vi "get iGPS result.vi"(8 "error in":errorcluster, 10 "serial number":string, 11 "PLC Comms":T3={"PLC boolean read Tags"={"AT glass position"={"Tag Name"="S060.PXI.Signals.PlltData.SN", "Network Path"="172.15.51.1,1,0", "use opc"=FALSE, "DataSocket Reference"={"CWDSLib._DCWDataSocket"=refnum, "CWDSLib._DCWData"=refnum, "OnDataUpdated"=0, "OnStatusUpdated"=0}}, "AT shade position"={"Tag Name"="S060.PXI.Signals.PlltData.SN", "Network Path"="172.15.51.1,1,0", "use opc"=FALSE, "DataSocket Reference"={"CWDSLib._DCWDataSocket"=refnum, "CWDSLib._DCWData"=refnum, "OnDataUpdated"=0, "OnStatusUpdated"=0}}, "AT in glass wand lower pos"={"Tag Name"="S060.PXI.Signals.PlltData.SN", "Network Path"="172.15.51.1,1,0", "use opc"=FALSE, "DataSocket Reference"={"CWDSLib._DCWDataSocket"=refnum, "CWDSLib._DCWData"=refnum, "OnDataUpdated"=0, "OnStatusUpdated"=0}}, "AT in sunshad wand lower pos"={"Tag Name"="S060.PXI.Signals.PlltData.SN", "Network Path"="172.15.51.1,1,0", "use opc"=FALSE, "DataSocket Reference"={"CWDSLib._DCWDataSocket"=refnum, "CWDSLib._DCWData"=refnum, "OnDataUpdated"=0, "OnStatusUpdated"=0}}, "AT in wand home pos"={"Tag Name"="S060.PXI.Signals.PlltData.SN", "Network Path"="172.15.51.1,1,0", "use opc"=FALSE, "DataSocket Reference"={"CWDSLib._DCWDataSocket"=refnum, "CWDSLib._DCWData"=refnum, "OnDataUpdated"=0, "OnStatusUpdated"=0}}, "LVDT's Extended"={"Tag Name"="S060.PXI.Signals.PlltData.SN", "Network Path"="172.15.51.1,1,0", "use opc"=FALSE, "DataSocket Reference"={"CWDSLib._DCWDataSocket"=refnum, "CWDSLib._DCWData"=refnum, "OnDataUpdated"=0, "OnStatusUpdated"=0}}, "bolt check 1"={"Tag Name"="S060.PXI.Signals.PlltData.SN", "Network Path"="172.15.51.1,1,0", "use opc"=FALSE, "DataSocket Reference"={"CWDSLib._DCWDataSocket"=refnum, "CWDSLib._DCWData"=refnum, "OnDataUpdated"=0, "OnStatusUpdated"=0}}, "bolt check 2"={"Tag Name"="S060.PXI.Signals.PlltData.SN", "Network Path"="172.15.51.1,1,0", "use opc"=FALSE, "DataSocket Reference"={"CWDSLib._DCWDataSocket"=refnum, "CWDSLib._DCWData"=refnum, "OnDataUpdated"=0, "OnStatusUpdated"=0}}, "bolt check 3"={"Tag Name"="S060.PXI.Signals.PlltData.SN", "Network Path"="172.15.51.1,1,0", "use opc"=FALSE, "DataSocket Reference"={"CWDSLib._DCWDataSocket"=refnum, "CWDSLib._DCWData"=refnum, "OnDataUpdated"=0, "OnStatusUpdated"=0}}, "bolt check 4"={"Tag Name"="S060.PXI.Signals.PlltData.SN", "Network Path"="172.15.51.1,1,0", "use opc"=FALSE, "DataSocket Reference"={"CWDSLib._DCWDataSocket"=refnum, "CWDSLib._DCWData"=refnum, "OnDataUpdated"=0, "OnStatusUpdated"=0}}, "bolt check 5"={"Tag Name"="S060.PXI.Signals.PlltData.SN", "Network Path"="172.15.51.1,1,0", "use opc"=FALSE, "DataSocket Reference"={"CWDSLib._DCWDataSocket"=refnum, "CWDSLib._DCWData"=refnum, "OnDataUpdated"=0, "OnStatusUpdated"=0}}, "bolt check 6"={"Tag Name"="S060.PXI.Signals.PlltData.SN", "Network Path"="172.15.51.1,1,0", "use opc"=FALSE, "DataSocket Reference"={"CWDSLib._DCWDataSocket"=refnum, "CWDSLib._DCWData"=refnum, "OnDataUpdated"=0, "OnStatusUpdated"=0}}, "bolt check 7"={"Tag Name"="S060.PXI.Signals.PlltData.SN", "Network Path"="172.15.51.1,1,0", "use opc"=FALSE, "DataSocket Reference"={"CWDSLib._DCWDataSocket"=refnum, "CWDSLib._DCWData"=refnum, "OnDataUpdated"=0, "OnStatusUpdated"=0}}, "bolt check 8"={"Tag Name"="S060.PXI.Signals.PlltData.SN", "Network Path"="172.15.51.1,1,0", "use opc"=FALSE, "DataSocket Reference"={"CWDSLib._DCWDataSocket"=refnum, "CWDSLib._DCWData"=refnum, "OnDataUpdated"=0, "OnStatusUpdated"=0}}, "start"={"Tag Name"="S060.PXI.Signals.PlltData.SN", "Network Path"="172.15.51.1,1,0", "use opc"=FALSE, "DataSocket Reference"={"CWDSLib._DCWDataSocket"=refnum, "CWDSLib._DCWData"=refnum, "OnDataUpdated"=0, "OnStatusUpdated"=0}}, "abort"={"Tag Name"="S060.PXI.Signals.PlltData.SN", "Network Path"="172.15.51.1,1,0", "use opc"=FALSE, "DataSocket Reference"={"CWDSLib._DCWDataSocket"=refnum, "CWDSLib._DCWData"=refnum, "OnDataUpdated"=0, "OnStatusUpdated"=0}}, "LVDT's Retracted"={"Tag Name"="S060.PXI.Signals.PlltData.SN", "Network Path"="172.15.51.1,1,0", "use opc"=FALSE, "DataSocket Reference"={"CWDSLib._DCWDataSocket"=refnum, "CWDSLib._DCWData"=refnum, "OnDataUpdated"=0, "OnStatusUpdated"=0}}, "manual barcode print"={"Tag Name"="S060.PXI.Signals.PlltData.SN", "Network Path"="172.15.51.1,1,0", "use opc"=FALSE, "DataSocket Reference"={"CWDSLib._DCWDataSocket"=refnum, "CWDSLib._DCWData"=refnum, "OnDataUpdated"=0, "OnStatusUpdated"=0}}, "ss servo at open"={"Tag Name"="S060.PXI.Signals.PlltData.SN", "Network Path"="172.15.51.1,1,0", "use opc"=FALSE, "DataSocket Reference"={"CWDSLib._DCWDataSocket"=refnum, "CWDSLib._DCWData"=refnum, "OnDataUpdated"=0, "OnStatusUpdated"=0}}, "ss servo at close"={"Tag Name"="S060.PXI.Signals.PlltData.SN", "Network Path"="172.15.51.1,1,0", "use opc"=FALSE, "DataSocket Reference"={"CWDSLib._DCWDataSocket"=refnum, "CWDSLib._DCWData"=refnum, "OnDataUpdated"=0, "OnStatusUpdated"=0}}, "ss servo opening"={"Tag Name"="S060.PXI.Signals.PlltData.SN", "Network Path"="172.15.51.1,1,0", "use opc"=FALSE, "DataSocket Reference"={"CWDSLib._DCWDataSocket"=refnum, "CWDSLib._DCWData"=refnum, "OnDataUpdated"=0, "OnStatusUpdated"=0}}, "ss servo closing"={"Tag Name"="S060.PXI.Signals.PlltData.SN", "Network Path"="172.15.51.1,1,0", "use opc"=FALSE, "DataSocket Reference"={"CWDSLib._DCWDataSocket"=refnum, "CWDSLib._DCWData"=refnum, "OnDataUpdated"=0, "OnStatusUpdated"=0}}, "control slide at home"={"Tag Name"="S060.PXI.Signals.PlltData.SN", "Network Path"="172.15.51.1,1,0", "use opc"=FALSE, "DataSocket Reference"={"CWDSLib._DCWDataSocket"=refnum, "CWDSLib._DCWData"=refnum, "OnDataUpdated"=0, "OnStatusUpdated"=0}}, "control slide left good"={"Tag Name"="S060.PXI.Signals.PlltData.SN", "Network Path"="172.15.51.1,1,0", "use opc"=FALSE, "DataSocket Reference"={"CWDSLib._DCWDataSocket"=refnum, "CWDSLib._DCWData"=refnum, "OnDataUpdated"=0, "OnStatusUpdated"=0}}, "control slide left over stroke"={"Tag Name"="S060.PXI.Signals.PlltData.SN", "Network Path"="172.15.51.1,1,0", "use opc"=FALSE, "DataSocket Reference"={"CWDSLib._DCWDataSocket"=refnum, "CWDSLib._DCWData"=refnum, "OnDataUpdated"=0, "OnStatusUpdated"=0}}, "control slide right good"={"Tag Name"="S060.PXI.Signals.PlltData.SN", "Network Path"="172.15.51.1,1,0", "use opc"=FALSE, "DataSocket Reference"={"CWDSLib._DCWDataSocket"=refnum, "CWDSLib._DCWData"=refnum, "OnDataUpdated"=0, "OnStatusUpdated"=0}}, "control slide right over stroke"={"Tag Name"="S060.PXI.Signals.PlltData.SN", "Network Path"="172.15.51.1,1,0", "use opc"=FALSE, "DataSocket Reference"={"CWDSLib._DCWDataSocket"=refnum, "CWDSLib._DCWData"=refnum, "OnDataUpdated"=0, "OnStatusUpdated"=0}}, "wind deflector high speed pos"={"Tag Name"="S060.PXI.Signals.PlltData.SN", "Network Path"="172.15.51.1,1,0", "use opc"=FALSE, "DataSocket Reference"={"CWDSLib._DCWDataSocket"=refnum, "CWDSLib._DCWData"=refnum, "OnDataUpdated"=0, "OnStatusUpdated"=0}}, "wind deflector low speed pos"={"Tag Name"="S060.PXI.Signals.PlltData.SN", "Network Path"="172.15.51.1,1,0", "use opc"=FALSE, "DataSocket Reference"={"CWDSLib._DCWDataSocket"=refnum, "CWDSLib._DCWData"=refnum, "OnDataUpdated"=0, "OnStatusUpdated"=0}}, "AT VentPMACatHome"={"Tag Name"="S060.PXI.Signals.PlltData.SN", "Network Path"="172.15.51.1,1,0", "use opc"=FALSE, "DataSocket Reference"={"CWDSLib._DCWDataSocket"=refnum, "CWDSLib._DCWData"=refnum, "OnDataUpdated"=0, "OnStatusUpdated"=0}}, "AT VentPMACisExtend"={"Tag Name"="S060.PXI.Signals.PlltData.SN", "Network Path"="172.15.51.1,1,0", "use opc"=FALSE, "DataSocket Reference"={"CWDSLib._DCWDataSocket"=refnum, "CWDSLib._DCWData"=refnum, "OnDataUpdated"=0, "OnStatusUpdated"=0}}, "SS Barcode Scanner Bypassed"={"Tag Name"="S060.PXI.Signals.PlltData.SN", "Network Path"="172.15.51.1,1,0", "use opc"=FALSE, "DataSocket Reference"={"CWDSLib._DCWDataSocket"=refnum, "CWDSLib._DCWData"=refnum, "OnDataUpdated"=0, "OnStatusUpdated"=0}}, "Check Frame Barcode"={"Tag Name"="S060.PXI.Signals.PlltData.SN", "Network Path"="172.15.51.1,1,0", "use opc"=FALSE, "DataSocket Reference"={"CWDSLib._DCWDataSocket"=refnum, "CWDSLib._DCWData"=refnum, "OnDataUpdated"=0, "OnStatusUpdated"=0}}, "Z LVDTs Extended"={"Tag Name"="S060.PXI.Signals.PlltData.SN", "Network Path"="172.15.51.1,1,0", "use opc"=FALSE, "DataSocket Reference"={"CWDSLib._DCWDataSocket"=refnum, "CWDSLib._DCWData"=refnum, "OnDataUpdated"=0, "OnStatusUpdated"=0}}, "NVH Operator Pass"={"Tag Name"="S060.PXI.Signals.PlltData.SN", "Network Path"="172.15.51.1,1,0", "use opc"=FALSE, "DataSocket Reference"={"CWDSLib._DCWDataSocket"=refnum, "CWDSLib._DCWData"=refnum, "OnDataUpdated"=0, "OnStatusUpdated"=0}}, "NVH Operator Fail"={"Tag Name"="S060.PXI.Signals.PlltData.SN", "Network Path"="172.15.51.1,1,0", "use opc"=FALSE, "DataSocket Reference"={"CWDSLib._DCWDataSocket"=refnum, "CWDSLib._DCWData"=refnum, "OnDataUpdated"=0, "OnStatusUpdated"=0}}, "NVH Operator Express Glass Open"={"Tag Name"="S060.PXI.Signals.PlltData.SN", "Network Path"="172.15.51.1,1,0", "use opc"=FALSE, "DataSocket Reference"={"CWDSLib._DCWDataSocket"=refnum, "CWDSLib._DCWData"=refnum, "OnDataUpdated"=0, "OnStatusUpdated"=0}}, "NVH Operator Express Glass Close"={"Tag Name"="S060.PXI.Signals.PlltData.SN", "Network Path"="172.15.51.1,1,0", "use opc"=FALSE, "DataSocket Reference"={"CWDSLib._DCWDataSocket"=refnum, "CWDSLib._DCWData"=refnum, "OnDataUpdated"=0, "OnStatusUpdated"=0}}, "NVH Operator Express Rollo Open01"={"Tag Name"="S060.PXI.Signals.PlltData.SN", "Network Path"="172.15.51.1,1,0", "use opc"=FALSE, "DataSocket Reference"={"CWDSLib._DCWDataSocket"=refnum, "CWDSLib._DCWData"=refnum, "OnDataUpdated"=0, "OnStatusUpdated"=0}}, "NVH Operator Express Rollo Close01"={"Tag Name"="S060.PXI.Signals.PlltData.SN", "Network Path"="172.15.51.1,1,0", "use opc"=FALSE, "DataSocket Reference"={"CWDSLib._DCWDataSocket"=refnum, "CWDSLib._DCWData"=refnum, "OnDataUpdated"=0, "OnStatusUpdated"=0}}, "NVH Operator Express Rollo Open02"={"Tag Name"="S060.PXI.Signals.PlltData.SN", "Network Path"="172.15.51.1,1,0", "use opc"=FALSE, "DataSocket Reference"={"CWDSLib._DCWDataSocket"=refnum, "CWDSLib._DCWData"=refnum, "OnDataUpdated"=0, "OnStatusUpdated"=0}}, "NVH Operator Express Rollo Close02"={"Tag Name"="S060.PXI.Signals.PlltData.SN", "Network Path"="172.15.51.1,1,0", "use opc"=FALSE, "DataSocket Reference"={"CWDSLib._DCWDataSocket"=refnum, "CWDSLib._DCWData"=refnum, "OnDataUpdated"=0, "OnStatusUpdated"=0}}, "NVH Operator Vent Open Noise"={"Tag Name"="S060.PXI.Signals.PlltData.SN", "Network Path"="172.15.51.1,1,0", "use opc"=FALSE, "DataSocket Reference"={"CWDSLib._DCWDataSocket"=refnum, "CWDSLib._DCWData"=refnum, "OnDataUpdated"=0, "OnStatusUpdated"=0}}, "NVH Operator Vent Close Noise"={"Tag Name"="S060.PXI.Signals.PlltData.SN", "Network Path"="172.15.51.1,1,0", "use opc"=FALSE, "DataSocket Reference"={"CWDSLib._DCWDataSocket"=refnum, "CWDSLib._DCWData"=refnum, "OnDataUpdated"=0, "OnStatusUpdated"=0}}, "NVH Operator Sunshade Open Noise"={"Tag Name"="S060.PXI.Signals.PlltData.SN", "Network Path"="172.15.51.1,1,0", "use opc"=FALSE, "DataSocket Reference"={"CWDSLib._DCWDataSocket"=refnum, "CWDSLib._DCWData"=refnum, "OnDataUpdated"=0, "OnStatusUpdated"=0}}, "NVH Operator Sunshade Close Noise"={"Tag Name"="S060.PXI.Signals.PlltData.SN", "Network Path"="172.15.51.1,1,0", "use opc"=FALSE, "DataSocket Reference"={"CWDSLib._DCWDataSocket"=refnum, "CWDSLib._DCWData"=refnum, "OnDataUpdated"=0, "OnStatusUpdated"=0}}, "NVH Operator Glass Open Noise"={"Tag Name"="S060.PXI.Signals.PlltData.SN", "Network Path"="172.15.51.1,1,0", "use opc"=FALSE, "DataSocket Reference"={"CWDSLib._DCWDataSocket"=refnum, "CWDSLib._DCWData"=refnum, "OnDataUpdated"=0, "OnStatusUpdated"=0}}, "NVH Operator Glass Close Noise"={"Tag Name"="S060.PXI.Signals.PlltData.SN", "Network Path"="172.15.51.1,1,0", "use opc"=FALSE, "DataSocket Reference"={"CWDSLib._DCWDataSocket"=refnum, "CWDSLib._DCWData"=refnum, "OnDataUpdated"=0, "OnStatusUpdated"=0}}, "NVH Operator Finish"={"Tag Name"="S060.PXI.Signals.PlltData.SN", "Network Path"="172.15.51.1,1,0", "use opc"=FALSE, "DataSocket Reference"={"CWDSLib._DCWDataSocket"=refnum, "CWDSLib._DCWData"=refnum, "OnDataUpdated"=0, "OnStatusUpdated"=0}}, "NVH Operator Check"={"Tag Name"="S060.PXI.Signals.PlltData.SN", "Network Path"="172.15.51.1,1,0", "use opc"=FALSE, "DataSocket Reference"={"CWDSLib._DCWDataSocket"=refnum, "CWDSLib._DCWData"=refnum, "OnDataUpdated"=0, "OnStatusUpdated"=0}}, "windproof position"={"Tag Name"="S060.PXI.Signals.PlltData.SN", "Network Path"="172.15.51.1,1,0", "use opc"=FALSE, "DataSocket Reference"={"CWDSLib._DCWDataSocket"=refnum, "CWDSLib._DCWData"=refnum, "OnDataUpdated"=0, "OnStatusUpdated"=0}}, "NVH Operator Express Glass vent Open"={"Tag Name"="S060.PXI.Signals.PlltData.SN", "Network Path"="172.15.51.1,1,0", "use opc"=FALSE, "DataSocket Reference"={"CWDSLib._DCWDataSocket"=refnum, "CWDSLib._DCWData"=refnum, "OnDataUpdated"=0, "OnStatusUpdated"=0}}, "NVH Operator Express Glass Vent Close"={"Tag Name"="S060.PXI.Signals.PlltData.SN", "Network Path"="172.15.51.1,1,0", "use opc"=FALSE, "DataSocket Reference"={"CWDSLib._DCWDataSocket"=refnum, "CWDSLib._DCWData"=refnum, "OnDataUpdated"=0, "OnStatusUpdated"=0}}, "NVH Operator Re-do"={"Tag Name"="S060.PXI.Signals.PlltData.SN", "Network Path"="172.15.51.1,1,0", "use opc"=FALSE, "DataSocket Reference"={"CWDSLib._DCWDataSocket"=refnum, "CWDSLib._DCWData"=refnum, "OnDataUpdated"=0, "OnStatusUpdated"=0}}, "AT at vent ATS test pos"={"Tag Name"="S060.PXI.Signals.PlltData.SN", "Network Path"="172.15.51.1,1,0", "use opc"=FALSE, "DataSocket Reference"={"CWDSLib._DCWDataSocket"=refnum, "CWDSLib._DCWData"=refnum, "OnDataUpdated"=0, "OnStatusUpdated"=0}}, "AT at vent ATS Home pos"={"Tag Name"="S060.PXI.Signals.PlltData.SN", "Network Path"="172.15.51.1,1,0", "use opc"=FALSE, "DataSocket Reference"={"CWDSLib._DCWDataSocket"=refnum, "CWDSLib._DCWData"=refnum, "OnDataUpdated"=0, "OnStatusUpdated"=0}}, "Start Adjust LVDT"={"Tag Name"="S060.PXI.Signals.PlltData.SN", "Network Path"="172.15.51.1,1,0", "use opc"=FALSE, "DataSocket Reference"={"CWDSLib._DCWDataSocket"=refnum, "CWDSLib._DCWData"=refnum, "OnDataUpdated"=0, "OnStatusUpdated"=0}}, "Finish Adjust LVDT"={"Tag Name"="S060.PXI.Signals.PlltData.SN", "Network Path"="172.15.51.1,1,0", "use opc"=FALSE, "DataSocket Reference"={"CWDSLib._DCWDataSocket"=refnum, "CWDSLib._DCWData"=refnum, "OnDataUpdated"=0, "OnStatusUpdated"=0}}}, "PLC bool write Tags"={"AT set glass wand lower"={"Tag Name"="S060.PXI.Signals.PlltData.SN", "Network Path"="172.15.51.1,1,0", "use opc"=FALSE, "DataSocket Reference"={"CWDSLib._DCWDataSocket"=refnum, "CWDSLib._DCWData"=refnum, "OnDataUpdated"=0, "OnStatusUpdated"=0}}, "AT set sunshade wand lower"={"Tag Name"="S060.PXI.Signals.PlltData.SN", "Network Path"="172.15.51.1,1,0", "use opc"=FALSE, "DataSocket Reference"={"CWDSLib._DCWDataSocket"=refnum, "CWDSLib._DCWData"=refnum, "OnDataUpdated"=0, "OnStatusUpdated"=0}}, "AT set wand home pos"={"Tag Name"="S060.PXI.Signals.PlltData.SN", "Network Path"="172.15.51.1,1,0", "use opc"=FALSE, "DataSocket Reference"={"CWDSLib._DCWDataSocket"=refnum, "CWDSLib._DCWData"=refnum, "OnDataUpdated"=0, "OnStatusUpdated"=0}}, "Test Complete Pass"={"Tag Name"="S060.PXI.Signals.PlltData.SN", "Network Path"="172.15.51.1,1,0", "use opc"=FALSE, "DataSocket Reference"={"CWDSLib._DCWDataSocket"=refnum, "CWDSLib._DCWData"=refnum, "OnDataUpdated"=0, "OnStatusUpdated"=0}}, "Test Complete Fail"={"Tag Name"="S060.PXI.Signals.PlltData.SN", "Network Path"="172.15.51.1,1,0", "use opc"=FALSE, "DataSocket Reference"={"CWDSLib._DCWDataSocket"=refnum, "CWDSLib._DCWData"=refnum, "OnDataUpdated"=0, "OnStatusUpdated"=0}}, "Test Started"={"Tag Name"="S060.PXI.Signals.PlltData.SN", "Network Path"="172.15.51.1,1,0", "use opc"=FALSE, "DataSocket Reference"={"CWDSLib._DCWDataSocket"=refnum, "CWDSLib._DCWData"=refnum, "OnDataUpdated"=0, "OnStatusUpdated"=0}}, "Retract LVDT's"={"Tag Name"="S060.PXI.Signals.PlltData.SN", "Network Path"="172.15.51.1,1,0", "use opc"=FALSE, "DataSocket Reference"={"CWDSLib._DCWDataSocket"=refnum, "CWDSLib._DCWData"=refnum, "OnDataUpdated"=0, "OnStatusUpdated"=0}}, "Extend LVDT's"={"Tag Name"="S060.PXI.Signals.PlltData.SN", "Network Path"="172.15.51.1,1,0", "use opc"=FALSE, "DataSocket Reference"={"CWDSLib._DCWDataSocket"=refnum, "CWDSLib._DCWData"=refnum, "OnDataUpdated"=0, "OnStatusUpdated"=0}}, "ss servo open"={"Tag Name"="S060.PXI.Signals.PlltData.SN", "Network Path"="172.15.51.1,1,0", "use opc"=FALSE, "DataSocket Reference"={"CWDSLib._DCWDataSocket"=refnum, "CWDSLib._DCWData"=refnum, "OnDataUpdated"=0, "OnStatusUpdated"=0}}, "ss servo close"={"Tag Name"="S060.PXI.Signals.PlltData.SN", "Network Path"="172.15.51.1,1,0", "use opc"=FALSE, "DataSocket Reference"={"CWDSLib._DCWDataSocket"=refnum, "CWDSLib._DCWData"=refnum, "OnDataUpdated"=0, "OnStatusUpdated"=0}}, "control slide start"={"Tag Name"="S060.PXI.Signals.PlltData.SN", "Network Path"="172.15.51.1,1,0", "use opc"=FALSE, "DataSocket Reference"={"CWDSLib._DCWDataSocket"=refnum, "CWDSLib._DCWData"=refnum, "OnDataUpdated"=0, "OnStatusUpdated"=0}}, "control slide stop"={"Tag Name"="S060.PXI.Signals.PlltData.SN", "Network Path"="172.15.51.1,1,0", "use opc"=FALSE, "DataSocket Reference"={"CWDSLib._DCWDataSocket"=refnum, "CWDSLib._DCWData"=refnum, "OnDataUpdated"=0, "OnStatusUpdated"=0}}, "AT VentPMACHome"={"Tag Name"="S060.PXI.Signals.PlltData.SN", "Network Path"="172.15.51.1,1,0", "use opc"=FALSE, "DataSocket Reference"={"CWDSLib._DCWDataSocket"=refnum, "CWDSLib._DCWData"=refnum, "OnDataUpdated"=0, "OnStatusUpdated"=0}}, "AT VentPMACExtended"={"Tag Name"="S060.PXI.Signals.PlltData.SN", "Network Path"="172.15.51.1,1,0", "use opc"=FALSE, "DataSocket Reference"={"CWDSLib._DCWDataSocket"=refnum, "CWDSLib._DCWData"=refnum, "OnDataUpdated"=0, "OnStatusUpdated"=0}}, "Good Frame Barcode"={"Tag Name"="S060.PXI.Signals.PlltData.SN", "Network Path"="172.15.51.1,1,0", "use opc"=FALSE, "DataSocket Reference"={"CWDSLib._DCWDataSocket"=refnum, "CWDSLib._DCWData"=refnum, "OnDataUpdated"=0, "OnStatusUpdated"=0}}, "Bad Frame Barcode"={"Tag Name"="S060.PXI.Signals.PlltData.SN", "Network Path"="172.15.51.1,1,0", "use opc"=FALSE, "DataSocket Reference"={"CWDSLib._DCWDataSocket"=refnum, "CWDSLib._DCWData"=refnum, "OnDataUpdated"=0, "OnStatusUpdated"=0}}, "Extend Z LVDTS"={"Tag Name"="S060.PXI.Signals.PlltData.SN", "Network Path"="172.15.51.1,1,0", "use opc"=FALSE, "DataSocket Reference"={"CWDSLib._DCWDataSocket"=refnum, "CWDSLib._DCWData"=refnum, "OnDataUpdated"=0, "OnStatusUpdated"=0}}, "NVH SunRoof Moving"={"Tag Name"="S060.PXI.Signals.PlltData.SN", "Network Path"="172.15.51.1,1,0", "use opc"=FALSE, "DataSocket Reference"={"CWDSLib._DCWDataSocket"=refnum, "CWDSLib._DCWData"=refnum, "OnDataUpdated"=0, "OnStatusUpdated"=0}}, "NVH SunRoof Stop"={"Tag Name"="S060.PXI.Signals.PlltData.SN", "Network Path"="172.15.51.1,1,0", "use opc"=FALSE, "DataSocket Reference"={"CWDSLib._DCWDataSocket"=refnum, "CWDSLib._DCWData"=refnum, "OnDataUpdated"=0, "OnStatusUpdated"=0}}, "NVH Pass"={"Tag Name"="S060.PXI.Signals.PlltData.SN", "Network Path"="172.15.51.1,1,0", "use opc"=FALSE, "DataSocket Reference"={"CWDSLib._DCWDataSocket"=refnum, "CWDSLib._DCWData"=refnum, "OnDataUpdated"=0, "OnStatusUpdated"=0}}, "NVH Fail"={"Tag Name"="S060.PXI.Signals.PlltData.SN", "Network Path"="172.15.51.1,1,0", "use opc"=FALSE, "DataSocket Reference"={"CWDSLib._DCWDataSocket"=refnum, "CWDSLib._DCWData"=refnum, "OnDataUpdated"=0, "OnStatusUpdated"=0}}, "NVH Operator Express Glass Opened"={"Tag Name"="S060.PXI.Signals.PlltData.SN", "Network Path"="172.15.51.1,1,0", "use opc"=FALSE, "DataSocket Reference"={"CWDSLib._DCWDataSocket"=refnum, "CWDSLib._DCWData"=refnum, "OnDataUpdated"=0, "OnStatusUpdated"=0}}, "NVH Operator Express Glass Closed"={"Tag Name"="S060.PXI.Signals.PlltData.SN", "Network Path"="172.15.51.1,1,0", "use opc"=FALSE, "DataSocket Reference"={"CWDSLib._DCWDataSocket"=refnum, "CWDSLib._DCWData"=refnum, "OnDataUpdated"=0, "OnStatusUpdated"=0}}, "NVH Operator Express Rollo Opened01"={"Tag Name"="S060.PXI.Signals.PlltData.SN", "Network Path"="172.15.51.1,1,0", "use opc"=FALSE, "DataSocket Reference"={"CWDSLib._DCWDataSocket"=refnum, "CWDSLib._DCWData"=refnum, "OnDataUpdated"=0, "OnStatusUpdated"=0}}, "NVH Operator Express Rollo Closed01"={"Tag Name"="S060.PXI.Signals.PlltData.SN", "Network Path"="172.15.51.1,1,0", "use opc"=FALSE, "DataSocket Reference"={"CWDSLib._DCWDataSocket"=refnum, "CWDSLib._DCWData"=refnum, "OnDataUpdated"=0, "OnStatusUpdated"=0}}, "NVH Operator Express Rollo Opened02"={"Tag Name"="S060.PXI.Signals.PlltData.SN", "Network Path"="172.15.51.1,1,0", "use opc"=FALSE, "DataSocket Reference"={"CWDSLib._DCWDataSocket"=refnum, "CWDSLib._DCWData"=refnum, "OnDataUpdated"=0, "OnStatusUpdated"=0}}, "NVH Operator Pass"={"Tag Name"="S060.PXI.Signals.PlltData.SN", "Network Path"="172.15.51.1,1,0", "use opc"=FALSE, "DataSocket Reference"={"CWDSLib._DCWDataSocket"=refnum, "CWDSLib._DCWData"=refnum, "OnDataUpdated"=0, "OnStatusUpdated"=0}}, "NVH Operator Fail"={"Tag Name"="S060.PXI.Signals.PlltData.SN", "Network Path"="172.15.51.1,1,0", "use opc"=FALSE, "DataSocket Reference"={"CWDSLib._DCWDataSocket"=refnum, "CWDSLib._DCWData"=refnum, "OnDataUpdated"=0, "OnStatusUpdated"=0}}, "NVH Operator Check"={"Tag Name"="S060.PXI.Signals.PlltData.SN", "Network Path"="172.15.51.1,1,0", "use opc"=FALSE, "DataSocket Reference"={"CWDSLib._DCWDataSocket"=refnum, "CWDSLib._DCWData"=refnum, "OnDataUpdated"=0, "OnStatusUpdated"=0}}, "NVH Operator Vent Open Noise"={"Tag Name"="S060.PXI.Signals.PlltData.SN", "Network Path"="172.15.51.1,1,0", "use opc"=FALSE, "DataSocket Reference"={"CWDSLib._DCWDataSocket"=refnum, "CWDSLib._DCWData"=refnum, "OnDataUpdated"=0, "OnStatusUpdated"=0}}, "NVH Operator Vent Close Noise"={"Tag Name"="S060.PXI.Signals.PlltData.SN", "Network Path"="172.15.51.1,1,0", "use opc"=FALSE, "DataSocket Reference"={"CWDSLib._DCWDataSocket"=refnum, "CWDSLib._DCWData"=refnum, "OnDataUpdated"=0, "OnStatusUpdated"=0}}, "NVH Operator Sunshade Open Noise"={"Tag Name"="S060.PXI.Signals.PlltData.SN", "Network Path"="172.15.51.1,1,0", "use opc"=FALSE, "DataSocket Reference"={"CWDSLib._DCWDataSocket"=refnum, "CWDSLib._DCWData"=refnum, "OnDataUpdated"=0, "OnStatusUpdated"=0}}, "NVH Operator Sunshade Close Noise"={"Tag Name"="S060.PXI.Signals.PlltData.SN", "Network Path"="172.15.51.1,1,0", "use opc"=FALSE, "DataSocket Reference"={"CWDSLib._DCWDataSocket"=refnum, "CWDSLib._DCWData"=refnum, "OnDataUpdated"=0, "OnStatusUpdated"=0}}, "NVH Operator Glass Open Noise"={"Tag Name"="S060.PXI.Signals.PlltData.SN", "Network Path"="172.15.51.1,1,0", "use opc"=FALSE, "DataSocket Reference"={"CWDSLib._DCWDataSocket"=refnum, "CWDSLib._DCWData"=refnum, "OnDataUpdated"=0, "OnStatusUpdated"=0}}, "NVH Operator Glass Close Noise"={"Tag Name"="S060.PXI.Signals.PlltData.SN", "Network Path"="172.15.51.1,1,0", "use opc"=FALSE, "DataSocket Reference"={"CWDSLib._DCWDataSocket"=refnum, "CWDSLib._DCWData"=refnum, "OnDataUpdated"=0, "OnStatusUpdated"=0}}, "NVH Operator Finish"={"Tag Name"="S060.PXI.Signals.PlltData.SN", "Network Path"="172.15.51.1,1,0", "use opc"=FALSE, "DataSocket Reference"={"CWDSLib._DCWDataSocket"=refnum, "CWDSLib._DCWData"=refnum, "OnDataUpdated"=0, "OnStatusUpdated"=0}}, "AT set sunshade 02 wand up"={"Tag Name"="S060.PXI.Signals.PlltData.SN", "Network Path"="172.15.51.1,1,0", "use opc"=FALSE, "DataSocket Reference"={"CWDSLib._DCWDataSocket"=refnum, "CWDSLib._DCWData"=refnum, "OnDataUpdated"=0, "OnStatusUpdated"=0}}, "AT set wand 02 home pos"={"Tag Name"="S060.PXI.Signals.PlltData.SN", "Network Path"="172.15.51.1,1,0", "use opc"=FALSE, "DataSocket Reference"={"CWDSLib._DCWDataSocket"=refnum, "CWDSLib._DCWData"=refnum, "OnDataUpdated"=0, "OnStatusUpdated"=0}}, "Barcode01 OK"={"Tag Name"="S060.PXI.Signals.PlltData.SN", "Network Path"="172.15.51.1,1,0", "use opc"=FALSE, "DataSocket Reference"={"CWDSLib._DCWDataSocket"=refnum, "CWDSLib._DCWData"=refnum, "OnDataUpdated"=0, "OnStatusUpdated"=0}}, "Barcode02 OK"={"Tag Name"="S060.PXI.Signals.PlltData.SN", "Network Path"="172.15.51.1,1,0", "use opc"=FALSE, "DataSocket Reference"={"CWDSLib._DCWDataSocket"=refnum, "CWDSLib._DCWData"=refnum, "OnDataUpdated"=0, "OnStatusUpdated"=0}}, "AT set to Vent ATS Test Pos"={"Tag Name"="S060.PXI.Signals.PlltData.SN", "Network Path"="172.15.51.1,1,0", "use opc"=FALSE, "DataSocket Reference"={"CWDSLib._DCWDataSocket"=refnum, "CWDSLib._DCWData"=refnum, "OnDataUpdated"=0, "OnStatusUpdated"=0}}, "AT set to Vent ATS Home Pos"={"Tag Name"="S060.PXI.Signals.PlltData.SN", "Network Path"="172.15.51.1,1,0", "use opc"=FALSE, "DataSocket Reference"={"CWDSLib._DCWDataSocket"=refnum, "CWDSLib._DCWData"=refnum, "OnDataUpdated"=0, "OnStatusUpdated"=0}}, "Move LVDT Adjust Station"={"Tag Name"="S060.PXI.Signals.PlltData.SN", "Network Path"="172.15.51.1,1,0", "use opc"=FALSE, "DataSocket Reference"={"CWDSLib._DCWDataSocket"=refnum, "CWDSLib._DCWData"=refnum, "OnDataUpdated"=0, "OnStatusUpdated"=0}}}, "PLC string read Tags"={"Serial Number"={"Tag Name"="S060.PXI.Signals.PlltData.SN", "Network Path"="172.15.51.1,1,0", "use opc"=FALSE, "DataSocket Reference"={"CWDSLib._DCWDataSocket"=refnum, "CWDSLib._DCWData"=refnum, "OnDataUpdated"=0, "OnStatusUpdated"=0}}, "Pallet Number"={"Tag Name"="S060.PXI.Signals.PlltData.SN", "Network Path"="172.15.51.1,1,0", "use opc"=FALSE, "DataSocket Reference"={"CWDSLib._DCWDataSocket"=refnum, "CWDSLib._DCWData"=refnum, "OnDataUpdated"=0, "OnStatusUpdated"=0}}, "Inalfa Part Number"={"Tag Name"="S060.PXI.Signals.PlltData.SN", "Network Path"="172.15.51.1,1,0", "use opc"=FALSE, "DataSocket Reference"={"CWDSLib._DCWDataSocket"=refnum, "CWDSLib._DCWData"=refnum, "OnDataUpdated"=0, "OnStatusUpdated"=0}}, "Shade Color"={"Tag Name"="S060.PXI.Signals.PlltData.SN", "Network Path"="172.15.51.1,1,0", "use opc"=FALSE, "DataSocket Reference"={"CWDSLib._DCWDataSocket"=refnum, "CWDSLib._DCWData"=refnum, "OnDataUpdated"=0, "OnStatusUpdated"=0}}, "Model Type"={"Tag Name"="S060.PXI.Signals.PlltData.SN", "Network Path"="172.15.51.1,1,0", "use opc"=FALSE, "DataSocket Reference"={"CWDSLib._DCWDataSocket"=refnum, "CWDSLib._DCWData"=refnum, "OnDataUpdated"=0, "OnStatusUpdated"=0}}, "Customer Number"={"Tag Name"="S060.PXI.Signals.PlltData.SN", "Network Path"="172.15.51.1,1,0", "use opc"=FALSE, "DataSocket Reference"={"CWDSLib._DCWDataSocket"=refnum, "CWDSLib._DCWData"=refnum, "OnDataUpdated"=0, "OnStatusUpdated"=0}}, "Part History Number"={"Tag Name"="S060.PXI.Signals.PlltData.SN", "Network Path"="172.15.51.1,1,0", "use opc"=FALSE, "DataSocket Reference"={"CWDSLib._DCWDataSocket"=refnum, "CWDSLib._DCWData"=refnum, "OnDataUpdated"=0, "OnStatusUpdated"=0}}, "Shade 1 Barcode"={"Tag Name"="S060.PXI.Signals.PlltData.SN", "Network Path"="172.15.51.1,1,0", "use opc"=FALSE, "DataSocket Reference"={"CWDSLib._DCWDataSocket"=refnum, "CWDSLib._DCWData"=refnum, "OnDataUpdated"=0, "OnStatusUpdated"=0}}, "Shade 2 Barcode"={"Tag Name"="S060.PXI.Signals.PlltData.SN", "Network Path"="172.15.51.1,1,0", "use opc"=FALSE, "DataSocket Reference"={"CWDSLib._DCWDataSocket"=refnum, "CWDSLib._DCWData"=refnum, "OnDataUpdated"=0, "OnStatusUpdated"=0}}, "Manual Serial Number"={"Tag Name"="S060.PXI.Signals.PlltData.SN", "Network Path"="172.15.51.1,1,0", "use opc"=FALSE, "DataSocket Reference"={"CWDSLib._DCWDataSocket"=refnum, "CWDSLib._DCWData"=refnum, "OnDataUpdated"=0, "OnStatusUpdated"=0}}, "Manual Inalfa Part Number"={"Tag Name"="S060.PXI.Signals.PlltData.SN", "Network Path"="172.15.51.1,1,0", "use opc"=FALSE, "DataSocket Reference"={"CWDSLib._DCWDataSocket"=refnum, "CWDSLib._DCWData"=refnum, "OnDataUpdated"=0, "OnStatusUpdated"=0}}, "Manual Shade Color"={"Tag Name"="S060.PXI.Signals.PlltData.SN", "Network Path"="172.15.51.1,1,0", "use opc"=FALSE, "DataSocket Reference"={"CWDSLib._DCWDataSocket"=refnum, "CWDSLib._DCWData"=refnum, "OnDataUpdated"=0, "OnStatusUpdated"=0}}, "Manual Model Type"={"Tag Name"="S060.PXI.Signals.PlltData.SN", "Network Path"="172.15.51.1,1,0", "use opc"=FALSE, "DataSocket Reference"={"CWDSLib._DCWDataSocket"=refnum, "CWDSLib._DCWData"=refnum, "OnDataUpdated"=0, "OnStatusUpdated"=0}}, "Manual Customer Number"={"Tag Name"="S060.PXI.Signals.PlltData.SN", "Network Path"="172.15.51.1,1,0", "use opc"=FALSE, "DataSocket Reference"={"CWDSLib._DCWDataSocket"=refnum, "CWDSLib._DCWData"=refnum, "OnDataUpdated"=0, "OnStatusUpdated"=0}}, "Manual Part History Number"={"Tag Name"="S060.PXI.Signals.PlltData.SN", "Network Path"="172.15.51.1,1,0", "use opc"=FALSE, "DataSocket Reference"={"CWDSLib._DCWDataSocket"=refnum, "CWDSLib._DCWData"=refnum, "OnDataUpdated"=0, "OnStatusUpdated"=0}}, "iGPS SN 0"={"Tag Name"="S060.PXI.Signals.PlltData.SN", "Network Path"="172.15.51.1,1,0", "use opc"=FALSE, "DataSocket Reference"={"CWDSLib._DCWDataSocket"=refnum, "CWDSLib._DCWData"=refnum, "OnDataUpdated"=0, "OnStatusUpdated"=0}}, "iGPS SN 1"={"Tag Name"="S060.PXI.Signals.PlltData.SN", "Network Path"="172.15.51.1,1,0", "use opc"=FALSE, "DataSocket Reference"={"CWDSLib._DCWDataSocket"=refnum, "CWDSLib._DCWData"=refnum, "OnDataUpdated"=0, "OnStatusUpdated"=0}}, "iGPS SN 2"={"Tag Name"="S060.PXI.Signals.PlltData.SN", "Network Path"="172.15.51.1,1,0", "use opc"=FALSE, "DataSocket Reference"={"CWDSLib._DCWDataSocket"=refnum, "CWDSLib._DCWData"=refnum, "OnDataUpdated"=0, "OnStatusUpdated"=0}}, "iGPS SN 3"={"Tag Name"="S060.PXI.Signals.PlltData.SN", "Network Path"="172.15.51.1,1,0", "use opc"=FALSE, "DataSocket Reference"={"CWDSLib._DCWDataSocket"=refnum, "CWDSLib._DCWData"=refnum, "OnDataUpdated"=0, "OnStatusUpdated"=0}}, "iGPS SN 4"={"Tag Name"="S060.PXI.Signals.PlltData.SN", "Network Path"="172.15.51.1,1,0", "use opc"=FALSE, "DataSocket Reference"={"CWDSLib._DCWDataSocket"=refnum, "CWDSLib._DCWData"=refnum, "OnDataUpdated"=0, "OnStatusUpdated"=0}}, "iGPS SN 5"={"Tag Name"="S060.PXI.Signals.PlltData.SN", "Network Path"="172.15.51.1,1,0", "use opc"=FALSE, "DataSocket Reference"={"CWDSLib._DCWDataSocket"=refnum, "CWDSLib._DCWData"=refnum, "OnDataUpdated"=0, "OnStatusUpdated"=0}}, "iGPS SN 6"={"Tag Name"="S060.PXI.Signals.PlltData.SN", "Network Path"="172.15.51.1,1,0", "use opc"=FALSE, "DataSocket Reference"={"CWDSLib._DCWDataSocket"=refnum, "CWDSLib._DCWData"=refnum, "OnDataUpdated"=0, "OnStatusUpdated"=0}}, "iGPS SN 7"={"Tag Name"="S060.PXI.Signals.PlltData.SN", "Network Path"="172.15.51.1,1,0", "use opc"=FALSE, "DataSocket Reference"={"CWDSLib._DCWDataSocket"=refnum, "CWDSLib._DCWData"=refnum, "OnDataUpdated"=0, "OnStatusUpdated"=0}}, "iGPS SN 8"={"Tag Name"="S060.PXI.Signals.PlltData.SN", "Network Path"="172.15.51.1,1,0", "use opc"=FALSE, "DataSocket Reference"={"CWDSLib._DCWDataSocket"=refnum, "CWDSLib._DCWData"=refnum, "OnDataUpdated"=0, "OnStatusUpdated"=0}}, "iGPS SN 9"={"Tag Name"="S060.PXI.Signals.PlltData.SN", "Network Path"="172.15.51.1,1,0", "use opc"=FALSE, "DataSocket Reference"={"CWDSLib._DCWDataSocket"=refnum, "CWDSLib._DCWData"=refnum, "OnDataUpdated"=0, "OnStatusUpdated"=0}}}, "PLC string write Tags"={"barcode station error"={"Tag Name"="S060.PXI.Signals.PlltData.SN", "Network Path"="172.15.51.1,1,0", "use opc"=FALSE, "DataSocket Reference"={"CWDSLib._DCWDataSocket"=refnum, "CWDSLib._DCWData"=refnum, "OnDataUpdated"=0, "OnStatusUpdated"=0}}, "error message 0"={"Tag Name"="S060.PXI.Signals.PlltData.SN", "Network Path"="172.15.51.1,1,0", "use opc"=FALSE, "DataSocket Reference"={"CWDSLib._DCWDataSocket"=refnum, "CWDSLib._DCWData"=refnum, "OnDataUpdated"=0, "OnStatusUpdated"=0}}, "error message 1"={"Tag Name"="S060.PXI.Signals.PlltData.SN", "Network Path"="172.15.51.1,1,0", "use opc"=FALSE, "DataSocket Reference"={"CWDSLib._DCWDataSocket"=refnum, "CWDSLib._DCWData"=refnum, "OnDataUpdated"=0, "OnStatusUpdated"=0}}, "error message 2"={"Tag Name"="S060.PXI.Signals.PlltData.SN", "Network Path"="172.15.51.1,1,0", "use opc"=FALSE, "DataSocket Reference"={"CWDSLib._DCWDataSocket"=refnum, "CWDSLib._DCWData"=refnum, "OnDataUpdated"=0, "OnStatusUpdated"=0}}, "error message 3"={"Tag Name"="S060.PXI.Signals.PlltData.SN", "Network Path"="172.15.51.1,1,0", "use opc"=FALSE, "DataSocket Reference"={"CWDSLib._DCWDataSocket"=refnum, "CWDSLib._DCWData"=refnum, "OnDataUpdated"=0, "OnStatusUpdated"=0}}, "error message 4"={"Tag Name"="S060.PXI.Signals.PlltData.SN", "Network Path"="172.15.51.1,1,0", "use opc"=FALSE, "DataSocket Reference"={"CWDSLib._DCWDataSocket"=refnum, "CWDSLib._DCWData"=refnum, "OnDataUpdated"=0, "OnStatusUpdated"=0}}, "error message 5"={"Tag Name"="S060.PXI.Signals.PlltData.SN", "Network Path"="172.15.51.1,1,0", "use opc"=FALSE, "DataSocket Reference"={"CWDSLib._DCWDataSocket"=refnum, "CWDSLib._DCWData"=refnum, "OnDataUpdated"=0, "OnStatusUpdated"=0}}, "error message 6"={"Tag Name"="S060.PXI.Signals.PlltData.SN", "Network Path"="172.15.51.1,1,0", "use opc"=FALSE, "DataSocket Reference"={"CWDSLib._DCWDataSocket"=refnum, "CWDSLib._DCWData"=refnum, "OnDataUpdated"=0, "OnStatusUpdated"=0}}, "error message 7"={"Tag Name"="S060.PXI.Signals.PlltData.SN", "Network Path"="172.15.51.1,1,0", "use opc"=FALSE, "DataSocket Reference"={"CWDSLib._DCWDataSocket"=refnum, "CWDSLib._DCWData"=refnum, "OnDataUpdated"=0, "OnStatusUpdated"=0}}, "error message 8"={"Tag Name"="S060.PXI.Signals.PlltData.SN", "Network Path"="172.15.51.1,1,0", "use opc"=FALSE, "DataSocket Reference"={"CWDSLib._DCWDataSocket"=refnum, "CWDSLib._DCWData"=refnum, "OnDataUpdated"=0, "OnStatusUpdated"=0}}, "error message 9"={"Tag Name"="S060.PXI.Signals.PlltData.SN", "Network Path"="172.15.51.1,1,0", "use opc"=FALSE, "DataSocket Reference"={"CWDSLib._DCWDataSocket"=refnum, "CWDSLib._DCWData"=refnum, "OnDataUpdated"=0, "OnStatusUpdated"=0}}}, "use opc"=FALSE, "PLC/OPC Path"="", "PLC float read Tags"={"iGPS float read tags"=[]}} {"PLC string write Tags"."error message 9"."DataSocket Reference"."OnStatusUpdated" format="%.0x"; "PLC string write Tags"."error message 9"."DataSocket Reference"."OnDataUpdated" format="%.0x"; "PLC string write Tags"."error message 8"."DataSocket Reference"."OnStatusUpdated" format="%.0x"; "PLC string write Tags"."error message 8"."DataSocket Reference"."OnDataUpdated" format="%.0x"; "PLC string write Tags"."error message 7"."DataSocket Reference"."OnStatusUpdated" format="%.0x"; "PLC string write Tags"."error message 7"."DataSocket Reference"."OnDataUpdated" format="%.0x"; "PLC string write Tags"."error message 6"."DataSocket Reference"."OnStatusUpdated" format="%.0x"; "PLC string write Tags"."error message 6"."DataSocket Reference"."OnDataUpdated" format="%.0x"; "PLC string write Tags"."error message 5"."DataSocket Reference"."OnStatusUpdated" format="%.0x"; "PLC string write Tags"."error message 5"."DataSocket Reference"."OnDataUpdated" format="%.0x"; "PLC string write Tags"."error message 4"."DataSocket Reference"."OnStatusUpdated" format="%.0x"; "PLC string write Tags"."error message 4"."DataSocket Reference"."OnDataUpdated" format="%.0x"; "PLC string write Tags"."error message 3"."DataSocket Reference"."OnStatusUpdated" format="%.0x"; "PLC string write Tags"."error message 3"."DataSocket Reference"."OnDataUpdated" format="%.0x"; "PLC string write Tags"."error message 2"."DataSocket Reference"."OnStatusUpdated" format="%.0x"; "PLC string write Tags"."error message 2"."DataSocket Reference"."OnDataUpdated" format="%.0x"; "PLC string write Tags"."error message 1"."DataSocket Reference"."OnStatusUpdated" format="%.0x"; "PLC string write Tags"."error message 1"."DataSocket Reference"."OnDataUpdated" format="%.0x"; "PLC string write Tags"."error message 0"."DataSocket Reference"."OnStatusUpdated" format="%.0x"; "PLC string write Tags"."error message 0"."DataSocket Reference"."OnDataUpdated" format="%.0x"; "PLC string write Tags"."barcode station error"."DataSocket Reference"."OnStatusUpdated" format="%.0x"; "PLC string write Tags"."barcode station error"."DataSocket Reference"."OnDataUpdated" format="%.0x"; "PLC string read Tags"."iGPS SN 9"."DataSocket Reference"."OnStatusUpdated" format="%.0x"; "PLC string read Tags"."iGPS SN 9"."DataSocket Reference"."OnDataUpdated" format="%.0x"; "PLC string read Tags"."iGPS SN 8"."DataSocket Reference"."OnStatusUpdated" format="%.0x"; "PLC string read Tags"."iGPS SN 8"."DataSocket Reference"."OnDataUpdated" format="%.0x"; "PLC string read Tags"."iGPS SN 7"."DataSocket Reference"."OnStatusUpdated" format="%.0x"; "PLC string read Tags"."iGPS SN 7"."DataSocket Reference"."OnDataUpdated" format="%.0x"; "PLC string read Tags"."iGPS SN 6"."DataSocket Reference"."OnStatusUpdated" format="%.0x"; "PLC string read Tags"."iGPS SN 6"."DataSocket Reference"."OnDataUpdated" format="%.0x"; "PLC string read Tags"."iGPS SN 5"."DataSocket Reference"."OnStatusUpdated" format="%.0x"; "PLC string read Tags"."iGPS SN 5"."DataSocket Reference"."OnDataUpdated" format="%.0x"; "PLC string read Tags"."iGPS SN 4"."DataSocket Reference"."OnStatusUpdated" format="%.0x"; "PLC string read Tags"."iGPS SN 4"."DataSocket Reference"."OnDataUpdated" format="%.0x"; "PLC string read Tags"."iGPS SN 3"."DataSocket Reference"."OnStatusUpdated" format="%.0x"; "PLC string read Tags"."iGPS SN 3"."DataSocket Reference"."OnDataUpdated" format="%.0x"; "PLC string read Tags"."iGPS SN 2"."DataSocket Reference"."OnStatusUpdated" format="%.0x"; "PLC string read Tags"."iGPS SN 2"."DataSocket Reference"."OnDataUpdated" format="%.0x"; "PLC string read Tags"."iGPS SN 1"."DataSocket Reference"."OnStatusUpdated" format="%.0x"; "PLC string read Tags"."iGPS SN 1"."DataSocket Reference"."OnDataUpdated" format="%.0x"; "PLC string read Tags"."iGPS SN 0"."DataSocket Reference"."OnStatusUpdated" format="%.0x"; "PLC string read Tags"."iGPS SN 0"."DataSocket Reference"."OnDataUpdated" format="%.0x"; "PLC string read Tags"."Manual Part History Number"."DataSocket Reference"."OnStatusUpdated" format="%.0x"; "PLC string read Tags"."Manual Part History Number"."DataSocket Reference"."OnDataUpdated" format="%.0x"; "PLC string read Tags"."Manual Customer Number"."DataSocket Reference"."OnStatusUpdated" format="%.0x"; "PLC string read Tags"."Manual Customer Number"."DataSocket Reference"."OnDataUpdated" format="%.0x"; "PLC string read Tags"."Manual Model Type"."DataSocket Reference"."OnStatusUpdated" format="%.0x"; "PLC string read Tags"."Manual Model Type"."DataSocket Reference"."OnDataUpdated" format="%.0x"; "PLC string read Tags"."Manual Shade Color"."DataSocket Reference"."OnStatusUpdated" format="%.0x"; "PLC string read Tags"."Manual Shade Color"."DataSocket Reference"."OnDataUpdated" format="%.0x"; "PLC string read Tags"."Manual Inalfa Part Number"."DataSocket Reference"."OnStatusUpdated" format="%.0x"; "PLC string read Tags"."Manual Inalfa Part Number"."DataSocket Reference"."OnDataUpdated" format="%.0x"; "PLC string read Tags"."Manual Serial Number"."DataSocket Reference"."OnStatusUpdated" format="%.0x"; "PLC string read Tags"."Manual Serial Number"."DataSocket Reference"."OnDataUpdated" format="%.0x"; "PLC string read Tags"."Shade 2 Barcode"."DataSocket Reference"."OnStatusUpdated" format="%.0x"; "PLC string read Tags"."Shade 2 Barcode"."DataSocket Reference"."OnDataUpdated" format="%.0x"; "PLC string read Tags"."Shade 1 Barcode"."DataSocket Reference"."OnStatusUpdated" format="%.0x"; "PLC string read Tags"."Shade 1 Barcode"."DataSocket Reference"."OnDataUpdated" format="%.0x"; "PLC string read Tags"."Part History Number"."DataSocket Reference"."OnStatusUpdated" format="%.0x"; "PLC string read Tags"."Part History Number"."DataSocket Reference"."OnDataUpdated" format="%.0x"; "PLC string read Tags"."Customer Number"."DataSocket Reference"."OnStatusUpdated" format="%.0x"; "PLC string read Tags"."Customer Number"."DataSocket Reference"."OnDataUpdated" format="%.0x"; "PLC string read Tags"."Model Type"."DataSocket Reference"."OnStatusUpdated" format="%.0x"; "PLC string read Tags"."Model Type"."DataSocket Reference"."OnDataUpdated" format="%.0x"; "PLC string read Tags"."Shade Color"."DataSocket Reference"."OnStatusUpdated" format="%.0x"; "PLC string read Tags"."Shade Color"."DataSocket Reference"."OnDataUpdated" format="%.0x"; "PLC string read Tags"."Inalfa Part Number"."DataSocket Reference"."OnStatusUpdated" format="%.0x"; "PLC string read Tags"."Inalfa Part Number"."DataSocket Reference"."OnDataUpdated" format="%.0x"; "PLC string read Tags"."Pallet Number"."DataSocket Reference"."OnStatusUpdated" format="%.0x"; "PLC string read Tags"."Pallet Number"."DataSocket Reference"."OnDataUpdated" format="%.0x"; "PLC string read Tags"."Serial Number"."DataSocket Reference"."OnStatusUpdated" format="%.0x"; "PLC string read Tags"."Serial Number"."DataSocket Reference"."OnDataUpdated" format="%.0x"; "PLC bool write Tags"."Move LVDT Adjust Station"."DataSocket Reference"."OnStatusUpdated" format="%.0x"; "PLC bool write Tags"."Move LVDT Adjust Station"."DataSocket Reference"."OnDataUpdated" format="%.0x"; "PLC bool write Tags"."AT set to Vent ATS Home Pos"."DataSocket Reference"."OnStatusUpdated" format="%.0x"; "PLC bool write Tags"."AT set to Vent ATS Home Pos"."DataSocket Reference"."OnDataUpdated" format="%.0x"; "PLC bool write Tags"."AT set to Vent ATS Test Pos"."DataSocket Reference"."OnStatusUpdated" format="%.0x"; "PLC bool write Tags"."AT set to Vent ATS Test Pos"."DataSocket Reference"."OnDataUpdated" format="%.0x"; "PLC bool write Tags"."Barcode02 OK"."DataSocket Reference"."OnStatusUpdated" format="%.0x"; "PLC bool write Tags"."Barcode02 OK"."DataSocket Reference"."OnDataUpdated" format="%.0x"; "PLC bool write Tags"."Barcode01 OK"."DataSocket Reference"."OnStatusUpdated" format="%.0x"; "PLC bool write Tags"."Barcode01 OK"."DataSocket Reference"."OnDataUpdated" format="%.0x"; "PLC bool write Tags"."AT set wand 02 home pos"."DataSocket Reference"."OnStatusUpdated" format="%.0x"; "PLC bool write Tags"."AT set wand 02 home pos"."DataSocket Reference"."OnDataUpdated" format="%.0x"; "PLC bool write Tags"."AT set sunshade 02 wand up"."DataSocket Reference"."OnStatusUpdated" format="%.0x"; "PLC bool write Tags"."AT set sunshade 02 wand up"."DataSocket Reference"."OnDataUpdated" format="%.0x"; "PLC bool write Tags"."NVH Operator Finish"."DataSocket Reference"."OnStatusUpdated" format="%.0x"; "PLC bool write Tags"."NVH Operator Finish"."DataSocket Reference"."OnDataUpdated" format="%.0x"; "PLC bool write Tags"."NVH Operator Glass Close Noise"."DataSocket Reference"."OnStatusUpdated" format="%.0x"; "PLC bool write Tags"."NVH Operator Glass Close Noise"."DataSocket Reference"."OnDataUpdated" format="%.0x"; "PLC bool write Tags"."NVH Operator Glass Open Noise"."DataSocket Reference"."OnStatusUpdated" format="%.0x"; "PLC bool write Tags"."NVH Operator Glass Open Noise"."DataSocket Reference"."OnDataUpdated" format="%.0x"; "PLC bool write Tags"."NVH Operator Sunshade Close Noise"."DataSocket Reference"."OnStatusUpdated" format="%.0x"; "PLC bool write Tags"."NVH Operator Sunshade Close Noise"."DataSocket Reference"."OnDataUpdated" format="%.0x"; "PLC bool write Tags"."NVH Operator Sunshade Open Noise"."DataSocket Reference"."OnStatusUpdated" format="%.0x"; "PLC bool write Tags"."NVH Operator Sunshade Open Noise"."DataSocket Reference"."OnDataUpdated" format="%.0x"; "PLC bool write Tags"."NVH Operator Vent Close Noise"."DataSocket Reference"."OnStatusUpdated" format="%.0x"; "PLC bool write Tags"."NVH Operator Vent Close Noise"."DataSocket Reference"."OnDataUpdated" format="%.0x"; "PLC bool write Tags"."NVH Operator Vent Open Noise"."DataSocket Reference"."OnStatusUpdated" format="%.0x"; "PLC bool write Tags"."NVH Operator Vent Open Noise"."DataSocket Reference"."OnDataUpdated" format="%.0x"; "PLC bool write Tags"."NVH Operator Check"."DataSocket Reference"."OnStatusUpdated" format="%.0x"; "PLC bool write Tags"."NVH Operator Check"."DataSocket Reference"."OnDataUpdated" format="%.0x"; "PLC bool write Tags"."NVH Operator Fail"."DataSocket Reference"."OnStatusUpdated" format="%.0x"; "PLC bool write Tags"."NVH Operator Fail"."DataSocket Reference"."OnDataUpdated" format="%.0x"; "PLC bool write Tags"."NVH Operator Pass"."DataSocket Reference"."OnStatusUpdated" format="%.0x"; "PLC bool write Tags"."NVH Operator Pass"."DataSocket Reference"."OnDataUpdated" format="%.0x"; "PLC bool write Tags"."NVH Operator Express Rollo Opened02"."DataSocket Reference"."OnStatusUpdated" format="%.0x"; "PLC bool write Tags"."NVH Operator Express Rollo Opened02"."DataSocket Reference"."OnDataUpdated" format="%.0x"; "PLC bool write Tags"."NVH Operator Express Rollo Closed01"."DataSocket Reference"."OnStatusUpdated" format="%.0x"; "PLC bool write Tags"."NVH Operator Express Rollo Closed01"."DataSocket Reference"."OnDataUpdated" format="%.0x"; "PLC bool write Tags"."NVH Operator Express Rollo Opened01"."DataSocket Reference"."OnStatusUpdated" format="%.0x"; "PLC bool write Tags"."NVH Operator Express Rollo Opened01"."DataSocket Reference"."OnDataUpdated" format="%.0x"; "PLC bool write Tags"."NVH Operator Express Glass Closed"."DataSocket Reference"."OnStatusUpdated" format="%.0x"; "PLC bool write Tags"."NVH Operator Express Glass Closed"."DataSocket Reference"."OnDataUpdated" format="%.0x"; "PLC bool write Tags"."NVH Operator Express Glass Opened"."DataSocket Reference"."OnStatusUpdated" format="%.0x"; "PLC bool write Tags"."NVH Operator Express Glass Opened"."DataSocket Reference"."OnDataUpdated" format="%.0x"; "PLC bool write Tags"."NVH Fail"."DataSocket Reference"."OnStatusUpdated" format="%.0x"; "PLC bool write Tags"."NVH Fail"."DataSocket Reference"."OnDataUpdated" format="%.0x"; "PLC bool write Tags"."NVH Pass"."DataSocket Reference"."OnStatusUpdated" format="%.0x"; "PLC bool write Tags"."NVH Pass"."DataSocket Reference"."OnDataUpdated" format="%.0x"; "PLC bool write Tags"."NVH SunRoof Stop"."DataSocket Reference"."OnStatusUpdated" format="%.0x"; "PLC bool write Tags"."NVH SunRoof Stop"."DataSocket Reference"."OnDataUpdated" format="%.0x"; "PLC bool write Tags"."NVH SunRoof Moving"."DataSocket Reference"."OnStatusUpdated" format="%.0x"; "PLC bool write Tags"."NVH SunRoof Moving"."DataSocket Reference"."OnDataUpdated" format="%.0x"; "PLC bool write Tags"."Extend Z LVDTS"."DataSocket Reference"."OnStatusUpdated" format="%.0x"; "PLC bool write Tags"."Extend Z LVDTS"."DataSocket Reference"."OnDataUpdated" format="%.0x"; "PLC bool write Tags"."Bad Frame Barcode"."DataSocket Reference"."OnStatusUpdated" format="%.0x"; "PLC bool write Tags"."Bad Frame Barcode"."DataSocket Reference"."OnDataUpdated" format="%.0x"; "PLC bool write Tags"."Good Frame Barcode"."DataSocket Reference"."OnStatusUpdated" format="%.0x"; "PLC bool write Tags"."Good Frame Barcode"."DataSocket Reference"."OnDataUpdated" format="%.0x"; "PLC bool write Tags"."AT VentPMACExtended"."DataSocket Reference"."OnStatusUpdated" format="%.0x"; "PLC bool write Tags"."AT VentPMACExtended"."DataSocket Reference"."OnDataUpdated" format="%.0x"; "PLC bool write Tags"."AT VentPMACHome"."DataSocket Reference"."OnStatusUpdated" format="%.0x"; "PLC bool write Tags"."AT VentPMACHome"."DataSocket Reference"."OnDataUpdated" format="%.0x"; "PLC bool write Tags"."control slide stop"."DataSocket Reference"."OnStatusUpdated" format="%.0x"; "PLC bool write Tags"."control slide stop"."DataSocket Reference"."OnDataUpdated" format="%.0x"; "PLC bool write Tags"."control slide start"."DataSocket Reference"."OnStatusUpdated" format="%.0x"; "PLC bool write Tags"."control slide start"."DataSocket Reference"."OnDataUpdated" format="%.0x"; "PLC bool write Tags"."ss servo close"."DataSocket Reference"."OnStatusUpdated" format="%.0x"; "PLC bool write Tags"."ss servo close"."DataSocket Reference"."OnDataUpdated" format="%.0x"; "PLC bool write Tags"."ss servo open"."DataSocket Reference"."OnStatusUpdated" format="%.0x"; "PLC bool write Tags"."ss servo open"."DataSocket Reference"."OnDataUpdated" format="%.0x"; "PLC bool write Tags"."Extend LVDT's"."DataSocket Reference"."OnStatusUpdated" format="%.0x"; "PLC bool write Tags"."Extend LVDT's"."DataSocket Reference"."OnDataUpdated" format="%.0x"; "PLC bool write Tags"."Retract LVDT's"."DataSocket Reference"."OnStatusUpdated" format="%.0x"; "PLC bool write Tags"."Retract LVDT's"."DataSocket Reference"."OnDataUpdated" format="%.0x"; "PLC bool write Tags"."Test Started"."DataSocket Reference"."OnStatusUpdated" format="%.0x"; "PLC bool write Tags"."Test Started"."DataSocket Reference"."OnDataUpdated" format="%.0x"; "PLC bool write Tags"."Test Complete Fail"."DataSocket Reference"."OnStatusUpdated" format="%.0x"; "PLC bool write Tags"."Test Complete Fail"."DataSocket Reference"."OnDataUpdated" format="%.0x"; "PLC bool write Tags"."Test Complete Pass"."DataSocket Reference"."OnStatusUpdated" format="%.0x"; "PLC bool write Tags"."Test Complete Pass"."DataSocket Reference"."OnDataUpdated" format="%.0x"; "PLC bool write Tags"."AT set wand home pos"."DataSocket Reference"."OnStatusUpdated" format="%.0x"; "PLC bool write Tags"."AT set wand home pos"."DataSocket Reference"."OnDataUpdated" format="%.0x"; "PLC bool write Tags"."AT set sunshade wand lower"."DataSocket Reference"."OnStatusUpdated" format="%.0x"; "PLC bool write Tags"."AT set sunshade wand lower"."DataSocket Reference"."OnDataUpdated" format="%.0x"; "PLC bool write Tags"."AT set glass wand lower"."DataSocket Reference"."OnStatusUpdated" format="%.0x"; "PLC bool write Tags"."AT set glass wand lower"."DataSocket Reference"."OnDataUpdated" format="%.0x"; "PLC boolean read Tags"."Finish Adjust LVDT"."DataSocket Reference"."OnStatusUpdated" format="%.0x"; "PLC boolean read Tags"."Finish Adjust LVDT"."DataSocket Reference"."OnDataUpdated" format="%.0x"; "PLC boolean read Tags"."Start Adjust LVDT"."DataSocket Reference"."OnStatusUpdated" format="%.0x"; "PLC boolean read Tags"."Start Adjust LVDT"."DataSocket Reference"."OnDataUpdated" format="%.0x"; "PLC boolean read Tags"."AT at vent ATS Home pos"."DataSocket Reference"."OnStatusUpdated" format="%.0x"; "PLC boolean read Tags"."AT at vent ATS Home pos"."DataSocket Reference"."OnDataUpdated" format="%.0x"; "PLC boolean read Tags"."AT at vent ATS test pos"."DataSocket Reference"."OnStatusUpdated" format="%.0x"; "PLC boolean read Tags"."AT at vent ATS test pos"."DataSocket Reference"."OnDataUpdated" format="%.0x"; "PLC boolean read Tags"."NVH Operator Re-do"."DataSocket Reference"."OnStatusUpdated" format="%.0x"; "PLC boolean read Tags"."NVH Operator Re-do"."DataSocket Reference"."OnDataUpdated" format="%.0x"; "PLC boolean read Tags"."NVH Operator Express Glass Vent Close"."DataSocket Reference"."OnStatusUpdated" format="%.0x"; "PLC boolean read Tags"."NVH Operator Express Glass Vent Close"."DataSocket Reference"."OnDataUpdated" format="%.0x"; "PLC boolean read Tags"."NVH Operator Express Glass vent Open"."DataSocket Reference"."OnStatusUpdated" format="%.0x"; "PLC boolean read Tags"."NVH Operator Express Glass vent Open"."DataSocket Reference"."OnDataUpdated" format="%.0x"; "PLC boolean read Tags"."windproof position"."DataSocket Reference"."OnStatusUpdated" format="%.0x"; "PLC boolean read Tags"."windproof position"."DataSocket Reference"."OnDataUpdated" format="%.0x"; "PLC boolean read Tags"."NVH Operator Check"."DataSocket Reference"."OnStatusUpdated" format="%.0x"; "PLC boolean read Tags"."NVH Operator Check"."DataSocket Reference"."OnDataUpdated" format="%.0x"; "PLC boolean read Tags"."NVH Operator Finish"."DataSocket Reference"."OnStatusUpdated" format="%.0x"; "PLC boolean read Tags"."NVH Operator Finish"."DataSocket Reference"."OnDataUpdated" format="%.0x"; "PLC boolean read Tags"."NVH Operator Glass Close Noise"."DataSocket Reference"."OnStatusUpdated" format="%.0x"; "PLC boolean read Tags"."NVH Operator Glass Close Noise"."DataSocket Reference"."OnDataUpdated" format="%.0x"; "PLC boolean read Tags"."NVH Operator Glass Open Noise"."DataSocket Reference"."OnStatusUpdated" format="%.0x"; "PLC boolean read Tags"."NVH Operator Glass Open Noise"."DataSocket Reference"."OnDataUpdated" format="%.0x"; "PLC boolean read Tags"."NVH Operator Sunshade Close Noise"."DataSocket Reference"."OnStatusUpdated" format="%.0x"; "PLC boolean read Tags"."NVH Operator Sunshade Close Noise"."DataSocket Reference"."OnDataUpdated" format="%.0x"; "PLC boolean read Tags"."NVH Operator Sunshade Open Noise"."DataSocket Reference"."OnStatusUpdated" format="%.0x"; "PLC boolean read Tags"."NVH Operator Sunshade Open Noise"."DataSocket Reference"."OnDataUpdated" format="%.0x"; "PLC boolean read Tags"."NVH Operator Vent Close Noise"."DataSocket Reference"."OnStatusUpdated" format="%.0x"; "PLC boolean read Tags"."NVH Operator Vent Close Noise"."DataSocket Reference"."OnDataUpdated" format="%.0x"; "PLC boolean read Tags"."NVH Operator Vent Open Noise"."DataSocket Reference"."OnStatusUpdated" format="%.0x"; "PLC boolean read Tags"."NVH Operator Vent Open Noise"."DataSocket Reference"."OnDataUpdated" format="%.0x"; "PLC boolean read Tags"."NVH Operator Express Rollo Close02"."DataSocket Reference"."OnStatusUpdated" format="%.0x"; "PLC boolean read Tags"."NVH Operator Express Rollo Close02"."DataSocket Reference"."OnDataUpdated" format="%.0x"; "PLC boolean read Tags"."NVH Operator Express Rollo Open02"."DataSocket Reference"."OnStatusUpdated" format="%.0x"; "PLC boolean read Tags"."NVH Operator Express Rollo Open02"."DataSocket Reference"."OnDataUpdated" format="%.0x"; "PLC boolean read Tags"."NVH Operator Express Rollo Close01"."DataSocket Reference"."OnStatusUpdated" format="%.0x"; "PLC boolean read Tags"."NVH Operator Express Rollo Close01"."DataSocket Reference"."OnDataUpdated" format="%.0x"; "PLC boolean read Tags"."NVH Operator Express Rollo Open01"."DataSocket Reference"."OnStatusUpdated" format="%.0x"; "PLC boolean read Tags"."NVH Operator Express Rollo Open01"."DataSocket Reference"."OnDataUpdated" format="%.0x"; "PLC boolean read Tags"."NVH Operator Express Glass Close"."DataSocket Reference"."OnStatusUpdated" format="%.0x"; "PLC boolean read Tags"."NVH Operator Express Glass Close"."DataSocket Reference"."OnDataUpdated" format="%.0x"; "PLC boolean read Tags"."NVH Operator Express Glass Open"."DataSocket Reference"."OnStatusUpdated" format="%.0x"; "PLC boolean read Tags"."NVH Operator Express Glass Open"."DataSocket Reference"."OnDataUpdated" format="%.0x"; "PLC boolean read Tags"."NVH Operator Fail"."DataSocket Reference"."OnStatusUpdated" format="%.0x"; "PLC boolean read Tags"."NVH Operator Fail"."DataSocket Reference"."OnDataUpdated" format="%.0x"; "PLC boolean read Tags"."NVH Operator Pass"."DataSocket Reference"."OnStatusUpdated" format="%.0x"; "PLC boolean read Tags"."NVH Operator Pass"."DataSocket Reference"."OnDataUpdated" format="%.0x"; "PLC boolean read Tags"."Z LVDTs Extended"."DataSocket Reference"."OnStatusUpdated" format="%.0x"; "PLC boolean read Tags"."Z LVDTs Extended"."DataSocket Reference"."OnDataUpdated" format="%.0x"; "PLC boolean read Tags"."Check Frame Barcode"."DataSocket Reference"."OnStatusUpdated" format="%.0x"; "PLC boolean read Tags"."Check Frame Barcode"."DataSocket Reference"."OnDataUpdated" format="%.0x"; "PLC boolean read Tags"."SS Barcode Scanner Bypassed"."DataSocket Reference"."OnStatusUpdated" format="%.0x"; "PLC boolean read Tags"."SS Barcode Scanner Bypassed"."DataSocket Reference"."OnDataUpdated" format="%.0x"; "PLC boolean read Tags"."AT VentPMACisExtend"."DataSocket Reference"."OnStatusUpdated" format="%.0x"; "PLC boolean read Tags"."AT VentPMACisExtend"."DataSocket Reference"."OnDataUpdated" format="%.0x"; "PLC boolean read Tags"."AT VentPMACatHome"."DataSocket Reference"."OnStatusUpdated" format="%.0x"; "PLC boolean read Tags"."AT VentPMACatHome"."DataSocket Reference"."OnDataUpdated" format="%.0x"; "PLC boolean read Tags"."wind deflector low speed pos"."DataSocket Reference"."OnStatusUpdated" format="%.0x"; "PLC boolean read Tags"."wind deflector low speed pos"."DataSocket Reference"."OnDataUpdated" format="%.0x"; "PLC boolean read Tags"."wind deflector high speed pos"."DataSocket Reference"."OnStatusUpdated" format="%.0x"; "PLC boolean read Tags"."wind deflector high speed pos"."DataSocket Reference"."OnDataUpdated" format="%.0x"; "PLC boolean read Tags"."control slide right over stroke"."DataSocket Reference"."OnStatusUpdated" format="%.0x"; "PLC boolean read Tags"."control slide right over stroke"."DataSocket Reference"."OnDataUpdated" format="%.0x"; "PLC boolean read Tags"."control slide right good"."DataSocket Reference"."OnStatusUpdated" format="%.0x"; "PLC boolean read Tags"."control slide right good"."DataSocket Reference"."OnDataUpdated" format="%.0x"; "PLC boolean read Tags"."control slide left over stroke"."DataSocket Reference"."OnStatusUpdated" format="%.0x"; "PLC boolean read Tags"."control slide left over stroke"."DataSocket Reference"."OnDataUpdated" format="%.0x"; "PLC boolean read Tags"."control slide left good"."DataSocket Reference"."OnStatusUpdated" format="%.0x"; "PLC boolean read Tags"."control slide left good"."DataSocket Reference"."OnDataUpdated" format="%.0x"; "PLC boolean read Tags"."control slide at home"."DataSocket Reference"."OnStatusUpdated" format="%.0x"; "PLC boolean read Tags"."control slide at home"."DataSocket Reference"."OnDataUpdated" format="%.0x"; "PLC boolean read Tags"."ss servo closing"."DataSocket Reference"."OnStatusUpdated" format="%.0x"; "PLC boolean read Tags"."ss servo closing"."DataSocket Reference"."OnDataUpdated" format="%.0x"; "PLC boolean read Tags"."ss servo opening"."DataSocket Reference"."OnStatusUpdated" format="%.0x"; "PLC boolean read Tags"."ss servo opening"."DataSocket Reference"."OnDataUpdated" format="%.0x"; "PLC boolean read Tags"."ss servo at close"."DataSocket Reference"."OnStatusUpdated" format="%.0x"; "PLC boolean read Tags"."ss servo at close"."DataSocket Reference"."OnDataUpdated" format="%.0x"; "PLC boolean read Tags"."ss servo at open"."DataSocket Reference"."OnStatusUpdated" format="%.0x"; "PLC boolean read Tags"."ss servo at open"."DataSocket Reference"."OnDataUpdated" format="%.0x"; "PLC boolean read Tags"."manual barcode print"."DataSocket Reference"."OnStatusUpdated" format="%.0x"; "PLC boolean read Tags"."manual barcode print"."DataSocket Reference"."OnDataUpdated" format="%.0x"; "PLC boolean read Tags"."LVDT's Retracted"."DataSocket Reference"."OnStatusUpdated" format="%.0x"; "PLC boolean read Tags"."LVDT's Retracted"."DataSocket Reference"."OnDataUpdated" format="%.0x"; "PLC boolean read Tags"."abort"."DataSocket Reference"."OnStatusUpdated" format="%.0x"; "PLC boolean read Tags"."abort"."DataSocket Reference"."OnDataUpdated" format="%.0x"; "PLC boolean read Tags"."start"."DataSocket Reference"."OnStatusUpdated" format="%.0x"; "PLC boolean read Tags"."start"."DataSocket Reference"."OnDataUpdated" format="%.0x"; "PLC boolean read Tags"."bolt check 8"."DataSocket Reference"."OnStatusUpdated" format="%.0x"; "PLC boolean read Tags"."bolt check 8"."DataSocket Reference"."OnDataUpdated" format="%.0x"; "PLC boolean read Tags"."bolt check 7"."DataSocket Reference"."OnStatusUpdated" format="%.0x"; "PLC boolean read Tags"."bolt check 7"."DataSocket Reference"."OnDataUpdated" format="%.0x"; "PLC boolean read Tags"."bolt check 6"."DataSocket Reference"."OnStatusUpdated" format="%.0x"; "PLC boolean read Tags"."bolt check 6"."DataSocket Reference"."OnDataUpdated" format="%.0x"; "PLC boolean read Tags"."bolt check 5"."DataSocket Reference"."OnStatusUpdated" format="%.0x"; "PLC boolean read Tags"."bolt check 5"."DataSocket Reference"."OnDataUpdated" format="%.0x"; "PLC boolean read Tags"."bolt check 4"."DataSocket Reference"."OnStatusUpdated" format="%.0x"; "PLC boolean read Tags"."bolt check 4"."DataSocket Reference"."OnDataUpdated" format="%.0x"; "PLC boolean read Tags"."bolt check 3"."DataSocket Reference"."OnStatusUpdated" format="%.0x"; "PLC boolean read Tags"."bolt check 3"."DataSocket Reference"."OnDataUpdated" format="%.0x"; "PLC boolean read Tags"."bolt check 2"."DataSocket Reference"."OnStatusUpdated" format="%.0x"; "PLC boolean read Tags"."bolt check 2"."DataSocket Reference"."OnDataUpdated" format="%.0x"; "PLC boolean read Tags"."bolt check 1"."DataSocket Reference"."OnStatusUpdated" format="%.0x"; "PLC boolean read Tags"."bolt check 1"."DataSocket Reference"."OnDataUpdated" format="%.0x"; "PLC boolean read Tags"."LVDT's Extended"."DataSocket Reference"."OnStatusUpdated" format="%.0x"; "PLC boolean read Tags"."LVDT's Extended"."DataSocket Reference"."OnDataUpdated" format="%.0x"; "PLC boolean read Tags"."AT in wand home pos"."DataSocket Reference"."OnStatusUpdated" format="%.0x"; "PLC boolean read Tags"."AT in wand home pos"."DataSocket Reference"."OnDataUpdated" format="%.0x"; "PLC boolean read Tags"."AT in sunshad wand lower pos"."DataSocket Reference"."OnStatusUpdated" format="%.0x"; "PLC boolean read Tags"."AT in sunshad wand lower pos"."DataSocket Reference"."OnDataUpdated" format="%.0x"; "PLC boolean read Tags"."AT in glass wand lower pos"."DataSocket Reference"."OnStatusUpdated" format="%.0x"; "PLC boolean read Tags"."AT in glass wand lower pos"."DataSocket Reference"."OnDataUpdated" format="%.0x"; "PLC boolean read Tags"."AT shade position"."DataSocket Reference"."OnStatusUpdated" format="%.0x"; "PLC boolean read Tags"."AT shade position"."DataSocket Reference"."OnDataUpdated" format="%.0x"; "PLC boolean read Tags"."AT glass position"."DataSocket Reference"."OnStatusUpdated" format="%.0x"; "PLC boolean read Tags"."AT glass position"."DataSocket Reference"."OnDataUpdated" format="%.0x"}) -> (0 "error out":errorcluster, 2 "found iGPS result":bool, 3 "iGPS overall results":T1)   [LabVIEW 2018]
uses:
  02.Type Def's/iGPS channel result.ctl
  02.Type Def's/iGPS overall results.ctl
  <vilib>/Platform/dataskt.llb/DataSocket Reference Type.ctl
  05.UserVI's/type defs/plc path and tag.ctl
  02.Type Def's/station plc read boolean tags.ctl
  02.Type Def's/station plc write boolean tags.ctl
  02.Type Def's/station plc read string tags.ctl
  02.Type Def's/station plc write string tags.ctl
  02.Type Def's/station plc read float tags.ctl
  02.Type Def's/plc comms params.ctl
  02.Type Def's/iGPS float tags.ctl
panel:
  # "start/abort only used by barcode instance, since there are discrete signals for this in the other stations."
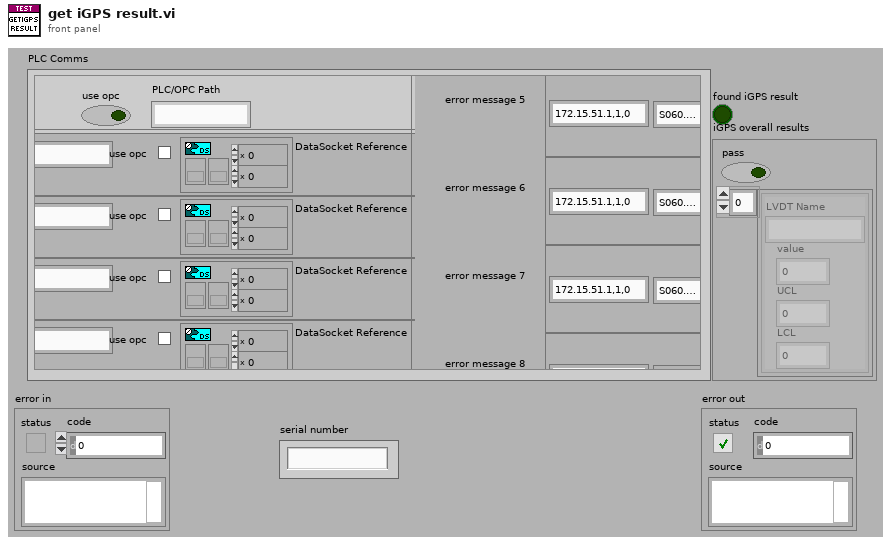
[diagram p1: front panel]
types:
  T1 = typedef "iGPS overall results.ctl" = cluster{"pass":bool, "channel results":T2[]}
  T2 = typedef "iGPS channel result.ctl" = cluster{"LVDT Name":string, "value":sgl, "UCL":sgl, "LCL":sgl}
  T3 = typedef "plc comms params.ctl" = cluster{"PLC boolean read Tags":T4, "PLC bool write Tags":T7, "PLC string read Tags":T8, "PLC string write Tags":T9, "use opc":bool, "PLC/OPC Path":string, "PLC float read Tags":T10}
  T4 = typedef "station plc read boolean tags.ctl" = cluster{"AT glass position":T5, "AT shade position":T5, "AT in glass wand lower pos":T5, "AT in sunshad wand lower pos":T5, "AT in wand home pos":T5, "LVDT's Extended":T5, "bolt check 1":T5, "bolt check 2":T5, "bolt check 3":T5, "bolt check 4":T5, "bolt check 5":T5, "bolt check 6":T5, "bolt check 7":T5, "bolt check 8":T5, "start":T5, "abort":T5, "LVDT's Retracted":T5, "manual barcode print":T5, "ss servo at open":T5, "ss servo at close":T5, "ss servo opening":T5, "ss servo closing":T5, "control slide at home":T5, "control slide left good":T5, "control slide left over stroke":T5, "control slide right good":T5, "control slide right over stroke":T5, "wind deflector high speed pos":T5, "wind deflector low speed pos":T5, "AT VentPMACatHome":T5, "AT VentPMACisExtend":T5, "SS Barcode Scanner Bypassed":T5, "Check Frame Barcode":T5, "Z LVDTs Extended":T5, "NVH Operator Pass":T5, "NVH Operator Fail":T5, "NVH Operator Express Glass Open":T5, "NVH Operator Express Glass Close":T5, "NVH Operator Express Rollo Open01":T5, "NVH Operator Express Rollo Close01":T5, "NVH Operator Express Rollo Open02":T5, "NVH Operator Express Rollo Close02":T5, "NVH Operator Vent Open Noise":T5, "NVH Operator Vent Close Noise":T5, "NVH Operator Sunshade Open Noise":T5, "NVH Operator Sunshade Close Noise":T5, "NVH Operator Glass Open Noise":T5, "NVH Operator Glass Close Noise":T5, "NVH Operator Finish":T5, "NVH Operator Check":T5, "windproof position":T5, "NVH Operator Express Glass vent Open":T5, "NVH Operator Express Glass Vent Close":T5, "NVH Operator Re-do":T5, "AT at vent ATS test pos":T5, "AT at vent ATS Home pos":T5, "Start Adjust LVDT":T5, "Finish Adjust LVDT":T5}
  T5 = typedef "plc path and tag.ctl" = cluster{"Tag Name":string, "Network Path":string, "use opc":bool, "DataSocket Reference":T6}
  T6 = typedef "DataSocket Reference Type.ctl" = cluster{"CWDSLib._DCWDataSocket":refnum<k7>, "CWDSLib._DCWData":refnum<k7>, "OnDataUpdated":u32, "OnStatusUpdated":u32}
  T7 = typedef "station plc write boolean tags.ctl" = cluster{"AT set glass wand lower":T5, "AT set sunshade wand lower":T5, "AT set wand home pos":T5, "Test Complete Pass":T5, "Test Complete Fail":T5, "Test Started":T5, "Retract LVDT's":T5, "Extend LVDT's":T5, "ss servo open":T5, "ss servo close":T5, "control slide start":T5, "control slide stop":T5, "AT VentPMACHome":T5, "AT VentPMACExtended":T5, "Good Frame Barcode":T5, "Bad Frame Barcode":T5, "Extend Z LVDTS":T5, "NVH SunRoof Moving":T5, "NVH SunRoof Stop":T5, "NVH Pass":T5, "NVH Fail":T5, "NVH Operator Express Glass Opened":T5, "NVH Operator Express Glass Closed":T5, "NVH Operator Express Rollo Opened01":T5, "NVH Operator Express Rollo Closed01":T5, "NVH Operator Express Rollo Opened02":T5, "NVH Operator Pass":T5, "NVH Operator Fail":T5, "NVH Operator Check":T5, "NVH Operator Vent Open Noise":T5, "NVH Operator Vent Close Noise":T5, "NVH Operator Sunshade Open Noise":T5, "NVH Operator Sunshade Close Noise":T5, "NVH Operator Glass Open Noise":T5, "NVH Operator Glass Close Noise":T5, "NVH Operator Finish":T5, "AT set sunshade 02 wand up":T5, "AT set wand 02 home pos":T5, "Barcode01 OK":T5, "Barcode02 OK":T5, "AT set to Vent ATS Test Pos":T5, "AT set to Vent ATS Home Pos":T5, "Move LVDT Adjust Station":T5}
  T8 = typedef "station plc read string tags.ctl" = cluster{"Serial Number":T5, "Pallet Number":T5, "Inalfa Part Number":T5, "Shade Color":T5, "Model Type":T5, "Customer Number":T5, "Part History Number":T5, "Shade 1 Barcode":T5, "Shade 2 Barcode":T5, "Manual Serial Number":T5, "Manual Inalfa Part Number":T5, "Manual Shade Color":T5, "Manual Model Type":T5, "Manual Customer Number":T5, "Manual Part History Number":T5, "iGPS SN 0":T5, "iGPS SN 1":T5, "iGPS SN 2":T5, "iGPS SN 3":T5, "iGPS SN 4":T5, "iGPS SN 5":T5, "iGPS SN 6":T5, "iGPS SN 7":T5, "iGPS SN 8":T5, "iGPS SN 9":T5}
  T9 = typedef "station plc write string tags.ctl" = cluster{"barcode station error":T5, "error message 0":T5, "error message 1":T5, "error message 2":T5, "error message 3":T5, "error message 4":T5, "error message 5":T5, "error message 6":T5, "error message 7":T5, "error message 8":T5, "error message 9":T5}
  T10 = typedef "station plc read float tags.ctl" = cluster{"iGPS float read tags":T11[]}
  T11 = typedef "iGPS float tags.ctl" = cluster{"LVDT measurements":cluster{"value":T5, "UCL":T5, "LCL":T5, "LVDT Name":string}[]}
  T12 = cluster{"value":T5, "UCL":T5, "LCL":T5, "LVDT Name":string}[]
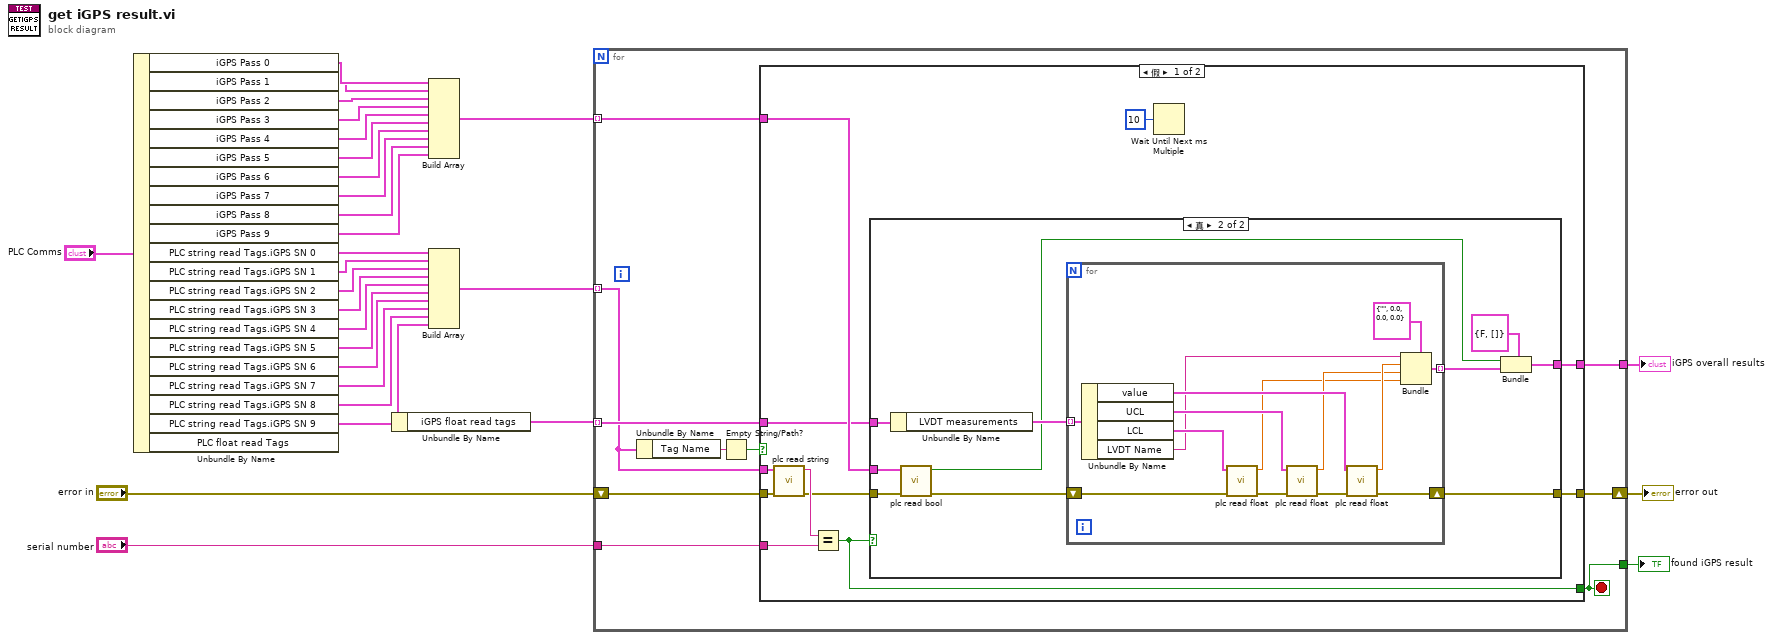
[diagram p0: block diagram]
diagram:
  n1 = Unbundle By Name("PLC Comms") -> ("iGPS Pass 0"=w27:T5, "iGPS Pass 1"=w26:T5, "iGPS Pass 2"=w25:T5, "iGPS Pass 3"=w24:T5, "iGPS Pass 4"=w23:T5, "iGPS Pass 5"=w22:T5, "iGPS Pass 6"=w21:T5, "iGPS Pass 7"=w20:T5, "iGPS Pass 8"=w19:T5, "iGPS Pass 9"=w18:T5, "PLC string read Tags.iGPS SN 0"=w17:T5, "PLC string read Tags.iGPS SN 1"=w16:T5, "PLC string read Tags.iGPS SN 2"=w15:T5, "PLC string read Tags.iGPS SN 3"=w14:T5, "PLC string read Tags.iGPS SN 4"=w13:T5, "PLC string read Tags.iGPS SN 5"=w12:T5, "PLC string read Tags.iGPS SN 6"=w11:T5, "PLC string read Tags.iGPS SN 7"=w10:T5, "PLC string read Tags.iGPS SN 8"=w9:T5, "PLC string read Tags.iGPS SN 9"=w8:T5, "PLC float read Tags"=w4:T10)
  n2 = Unbundle By Name(w4) -> ("iGPS float read tags"=w3:T11[])
  n3 = Build Array(w27, w26, w25, w24, w23, w22, w21, w20, w19, w18) -> (w5:T5[])
  n4 = Build Array(w17, w16, w15, w14, w13, w12, w11, w10, w9, w8) -> (w7:T5[])
  n5 = for {
    tunnel: w7 -> [w35] mode=indexing
    shift-right: [w37] -> w29
    shift-left: "error in" -> [w40]
    tunnel: "serial number" -> [w39]
    tunnel: w5 -> [w38] mode=indexing
    tunnel: w3 -> [w36] mode=indexing
    tunnel: [w32] -> w2
    tunnel: [w31] -> w1
    stop <- w31 stop-if-true
    n6 = Unbundle By Name(w35) -> ("Tag Name"=w34:string)
    n7 = Empty String/Path?(string/path=w34) -> (empty?=w33:bool)
    n8 = case shown="假" w33 {
      tunnel: w40 -> [w51 w77]
      tunnel: w39 -> [w49 _]
      tunnel: [w47 _] -> w31
      tunnel: w38 -> [w46 _]
      tunnel: [w44 w77] -> w37
      tunnel: w36 -> [w43 _]
      tunnel: w35 -> [w42 _]
      tunnel: [w41 _] -> w32
      frame False {
        n9 = call "plc read string.vi"("error in"=w51, "addr,tag"=w42) -> ("error out"=w45:errorcluster, "Data"=w48:string)  [unwired: 8 in]
        n10 = Equal?(x=w48, y=w49) -> (x = y?=w47:bool)
        n11 = case shown="真" w47 {
          tunnel: w46 -> [_ w62]
          tunnel: w45 -> [w52 w61]
          tunnel: [w52 w57] -> w44
          tunnel: w43 -> [_ w60]
          tunnel: [_ w53] -> w41
          frame False {
          }
          frame True {
            n12 = Unbundle By Name(w60) -> ("LVDT measurements"=w59:T12)
            n13 = call "plc read bool.vi"("error in"=w61, "addr,tag"=w62) -> ("error out"=w58:errorcluster, "value"=w55:bool)  [unwired: 8 in]
            n14 = for {
              tunnel: w59 -> [w76] mode=indexing
              shift-right: [w72] -> w57
              shift-left: w58 -> [w75]
              tunnel: [w63] -> w56 mode=indexing
              n15 = Unbundle By Name(w76) -> ("value"=w71:T5, "UCL"=w70:T5, "LCL"=w69:T5, "LVDT Name"=w68:string)
              n16 = call "plc read float.vi"("error in"=w75, "addr,tag"=w69) -> ("error out"=w74:errorcluster, "value"=w65:sgl)  [unwired: 8 in]
              n17 = call "plc read float.vi"("error in"=w74, "addr,tag"=w70) -> ("error out"=w73:errorcluster, "value"=w66:sgl)  [unwired: 8 in]
              n18 = call "plc read float.vi"("error in"=w73, "addr,tag"=w71) -> ("error out"=w72:errorcluster, "value"=w67:sgl)  [unwired: 8 in]
              n19 = Bundle(cluster=T2 {"LVDT Name"="", "value"=0.0, "UCL"=0.0, "LCL"=0.0}, "LVDT Name"=w68, "value"=w67, "UCL"=w66, "LCL"=w65) -> (w63:T2)
            }
            n20 = Bundle(cluster=T1 {"pass"=FALSE, "channel results"=[]}, "pass"=w55, "channel results"=w56) -> (w53:T1)
          }
        }
        n21 = Wait Until Next ms Multiple(millisecond multiple=u32 10) -> ()  [unwired: 1 out]
      }
      frame True {
      }
    }
  }
  "error out" <- w29
  "found iGPS result" <- w1
  "iGPS overall results" <- w2
